vi "Optionen Anzeige zum Speichern_Sicherungskopie.vi"(8 "Optionen":T1 {"SP laden speichern" items=["SP1"=1, "SP2"=2]; "Span Gas Auswahl" items=["1"=1, "2"=2, "3"=3, "4"=4, "5"=5, "6"=6, "7"=7, "8"=8]}, 10 "sichtbar":bool[](array[boolean]), 11 "Optionen (Eingang)":T3) -> (3 "Optionen (Ausgang)":T1 {"SP laden speichern" items=["SP1"=1, "SP2"=2]; "Span Gas Auswahl" items=["1"=1, "2"=2, "3"=3, "4"=4, "5"=5, "6"=6, "7"=7, "8"=8]})   [LabVIEW 2020]
uses:
  System Einstellungen/Optionen.ctl
  Funktionstasten/Spaneingang.ctl
  System Einstellungen/Optionen Eingabe.ctl
  Funktionstasten/Funktionstasten.lvlib
  System Einstellungen/System Einstellungen.lvlib
  System Einstellungen V2.lvlib
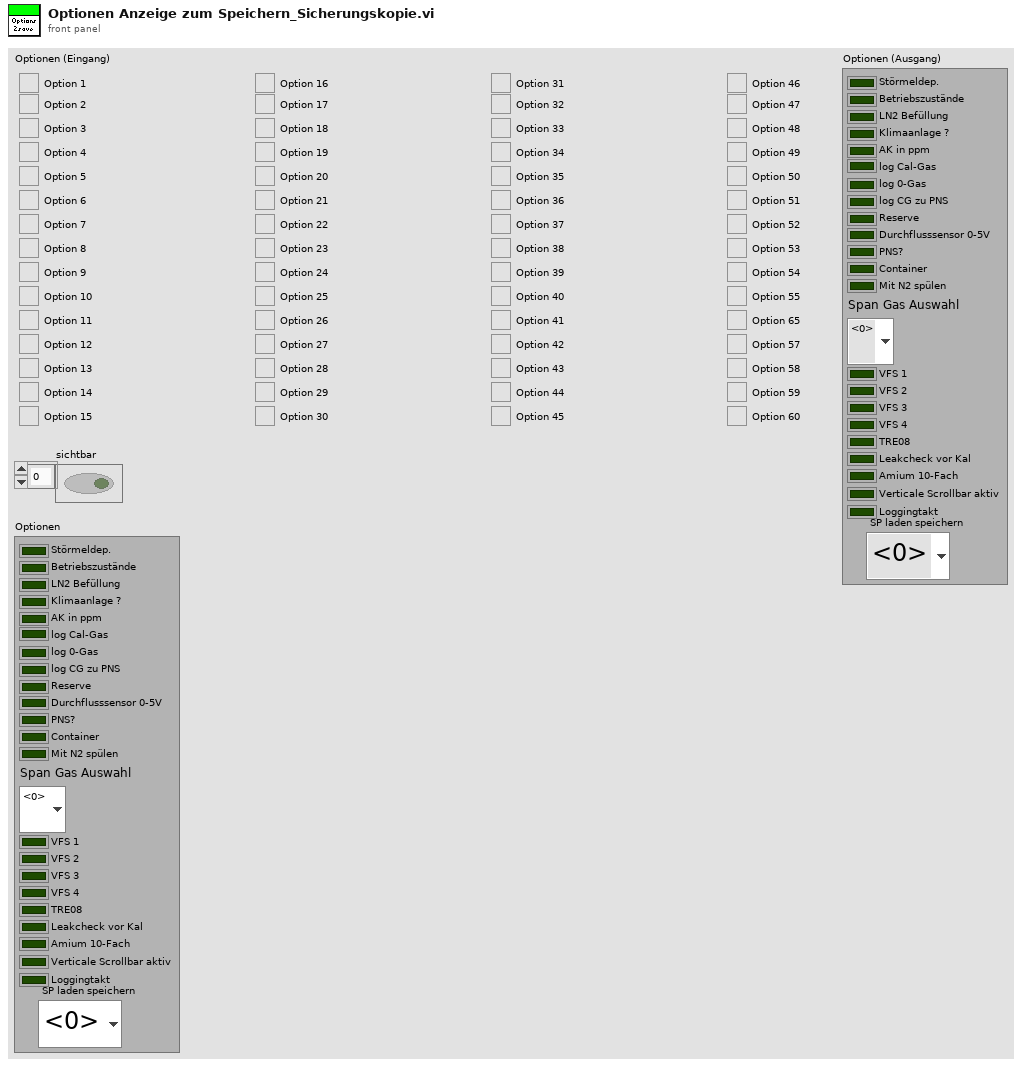
[diagram p1: front panel]
types:
  T1 = typedef "System Einstellungen.lvlib/Optionen.ctl" = cluster{"Störmeldep.":bool, "Betriebszustände":bool, "LN2 Befüllung":bool, "Klimaanlage ?":bool, "AK in ppm":bool, "log Cal-Gas":bool, "log 0-Gas":bool, "log CG zu PNS":bool, "Reserve":bool, "Durchflusssensor 0-5V":bool, "PNS?":bool, "Container":bool, "Mit N2 spülen":bool, "Span Gas Auswahl":T2, "VFS 1":bool, "VFS 2":bool, "VFS 3":bool, "VFS 4":bool, "TRE08":bool, "Leakcheck vor Kal":bool, "Amium 10-Fach":bool, "Verticale Scrollbar aktiv":bool, "Loggingtakt":bool, "SP laden speichern":u16}
  T2 = typedef "Funktionstasten.lvlib/Spaneingang.ctl" = u16
  T3 = typedef "System Einstellungen V2.lvlib/Optionen Eingabe.ctl" = cluster{"Option 1":bool, "Option 2":bool, "Option 3":bool, "Option 4":bool, "Option 5":bool, "Option 6":bool, "Option 7":bool, "Option 8":bool, "Option 9":bool, "Option 10":bool, "Option 11":bool, "Option 12":bool, "Option 13":bool, "Option 14":bool, "Option 15":bool, "Option 16":bool, "Option 17":bool, "Option 18":bool, "Option 19":bool, "Option 20":bool, "Option 21":bool, "Option 22":bool, "Option 23":bool, "Option 24":bool, "Option 25":bool, "Option 26":bool, "Option 27":bool, "Option 28":bool, "Option 29":bool, "Option 30":bool, "Option 31":bool, "Option 32":bool, "Option 33":bool, "Option 34":bool, "Option 35":bool, "Option 36":bool, "Option 37":bool, "Option 38":bool, "Option 39":bool, "Option 40":bool, "Option 41":bool, "Option 42":bool, "Option 43":bool, "Option 44":bool, "Option 45":bool, "Option 46":bool, "Option 47":bool, "Option 48":bool, "Option 49":bool, "Option 50":bool, "Option 51":bool, "Option 52":bool, "Option 53":bool, "Option 54":bool, "Option 55":bool, "Option 56":bool, "Option 57":bool, "Option 58":bool, "Option 59":bool, "Option 60":bool}
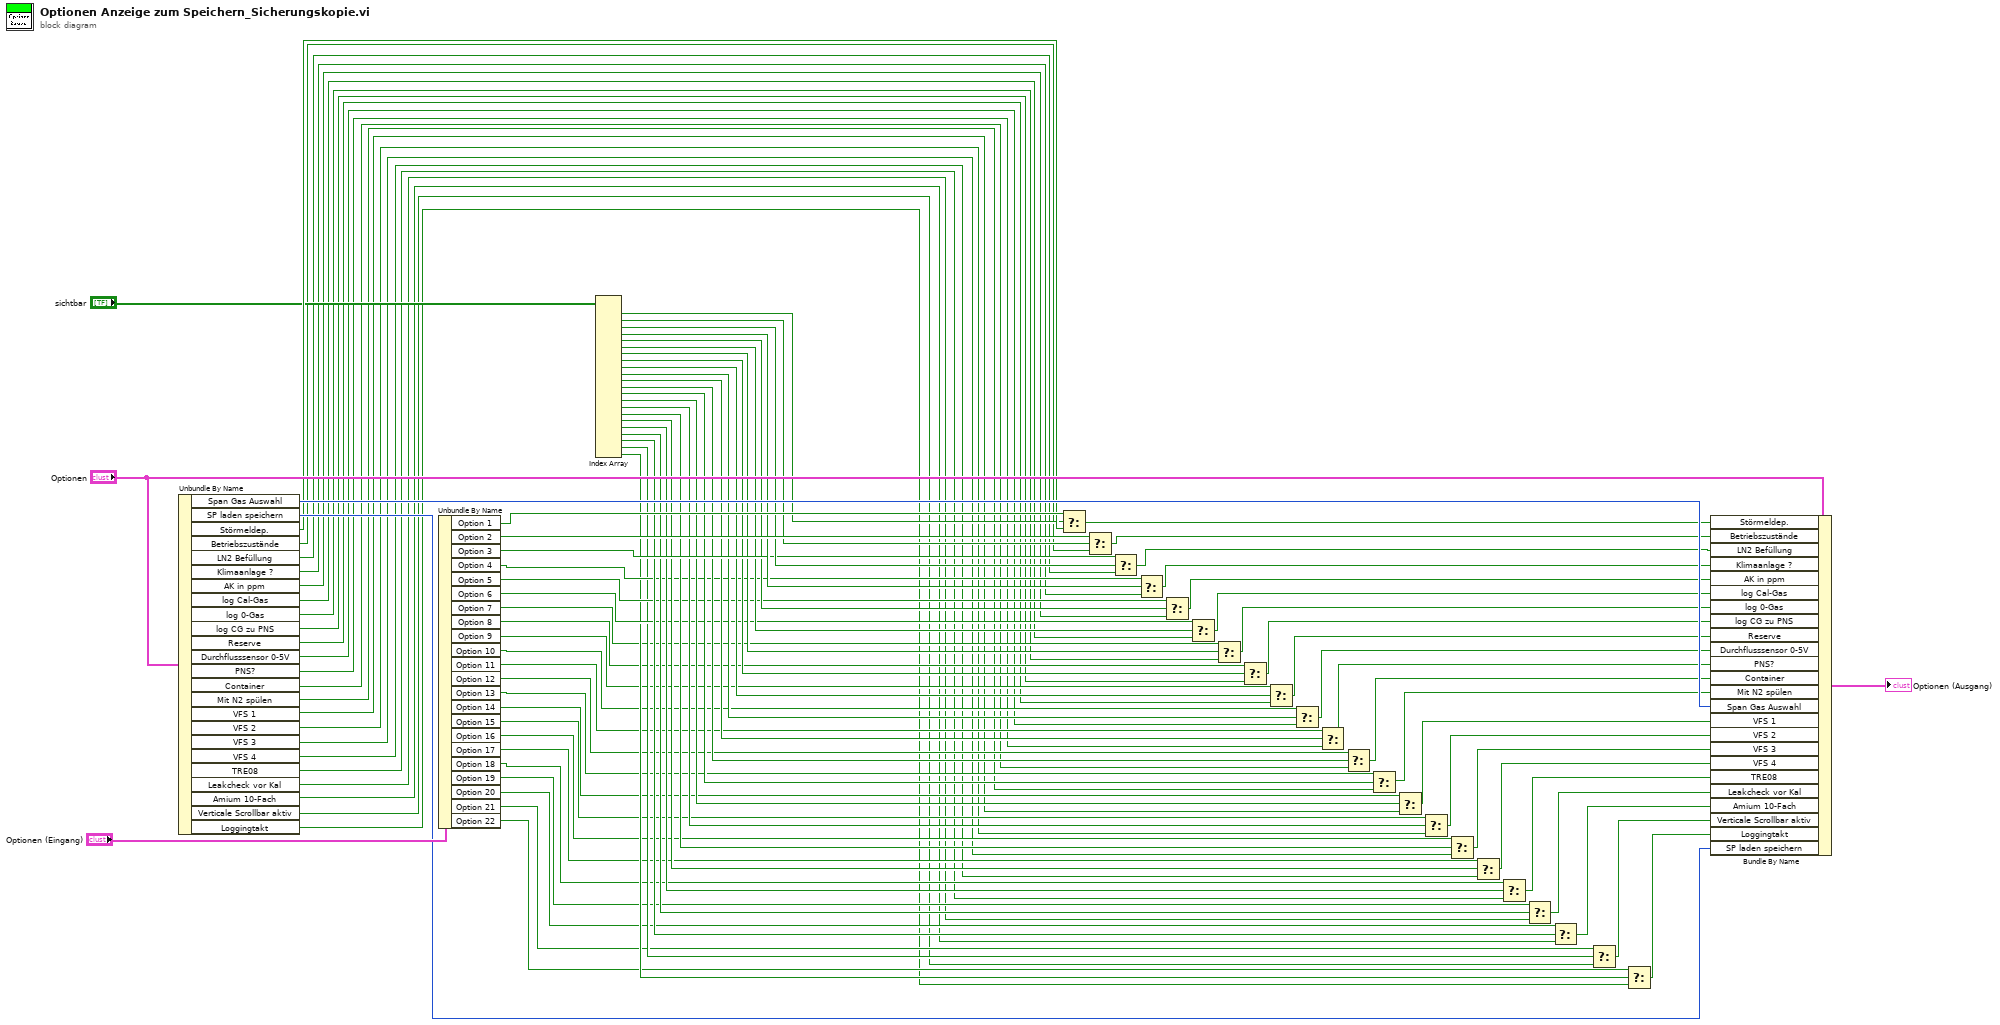
[diagram p0: block diagram]
diagram:
  n1 = Unbundle By Name("Optionen") -> ("Span Gas Auswahl"=w92:T2, "SP laden speichern"=w90:u16, "Störmeldep."=w87:bool, "Betriebszustände"=w11:bool, "LN2 Befüllung"=w78:bool, "Klimaanlage ?"=w58:bool, "AK in ppm"=w57:bool, "log Cal-Gas"=w12:bool, "log 0-Gas"=w33:bool, "log CG zu PNS"=w31:bool, "Reserve"=w29:bool, "Durchflusssensor 0-5V"=w27:bool, "PNS?"=w25:bool, "Container"=w23:bool, "Mit N2 spülen"=w10:bool, "VFS 1"=w9:bool, "VFS 2"=w8:bool, "VFS 3"=w7:bool, "VFS 4"=w6:bool, "TRE08"=w5:bool, "Leakcheck vor Kal"=w4:bool, "Amium 10-Fach"=w3:bool, "Verticale Scrollbar aktiv"=w2:bool, "Loggingtakt"=w1:bool)
  n2 = Unbundle By Name("Optionen (Eingang)") -> ("Option 1"=w88:bool, "Option 2"=w83:bool, "Option 3"=w79:bool, "Option 4"=w61:bool, "Option 5"=w60:bool, "Option 6"=w59:bool, "Option 7"=w34:bool, "Option 8"=w32:bool, "Option 9"=w30:bool, "Option 10"=w28:bool, "Option 11"=w26:bool, "Option 12"=w24:bool, "Option 13"=w22:bool, "Option 14"=w17:bool, "Option 15"=w21:bool, "Option 16"=w20:bool, "Option 17"=w19:bool, "Option 18"=w18:bool, "Option 19"=w16:bool, "Option 20"=w15:bool, "Option 21"=w14:bool, "Option 22"=w13:bool)
  n3 = Index Array(array="sichtbar") -> (element #1=w85:bool, element #2=w82:bool, element #3=w81:bool, element #4=w80:bool, element #5=w77:bool, element #6=w76:bool, element #7=w75:bool, element #8=w74:bool, element #9=w73:bool, element #10=w72:bool, element #11=w71:bool, element #12=w70:bool, element #13=w69:bool, element #14=w68:bool, element #15=w67:bool, element #16=w66:bool, element #17=w65:bool, element #18=w64:bool, element #19=w63:bool, element #20=w62:bool, element #21=w36:bool, element #22=w35:bool)  [unwired: 22 in]
  n4 = Select(t=w88, s=w85, f=w87) -> (s? t:f=w89:bool)
  n5 = Select(t=w83, s=w82, f=w11) -> (s? t:f=w84:bool)
  n6 = Select(t=w79, s=w81, f=w78) -> (s? t:f=w56:bool)
  n7 = Select(t=w61, s=w80, f=w58) -> (s? t:f=w55:bool)
  n8 = Select(t=w60, s=w77, f=w57) -> (s? t:f=w54:bool)
  n9 = Select(t=w59, s=w76, f=w12) -> (s? t:f=w53:bool)
  n10 = Select(t=w34, s=w75, f=w33) -> (s? t:f=w52:bool)
  n11 = Select(t=w32, s=w74, f=w31) -> (s? t:f=w51:bool)
  n12 = Select(t=w30, s=w73, f=w29) -> (s? t:f=w50:bool)
  n13 = Select(t=w28, s=w72, f=w27) -> (s? t:f=w49:bool)
  n14 = Select(t=w26, s=w71, f=w25) -> (s? t:f=w48:bool)
  n15 = Select(t=w24, s=w70, f=w23) -> (s? t:f=w47:bool)
  n16 = Select(t=w22, s=w69, f=w10) -> (s? t:f=w46:bool)
  n17 = Select(t=w17, s=w68, f=w9) -> (s? t:f=w45:bool)
  n18 = Select(t=w21, s=w67, f=w8) -> (s? t:f=w44:bool)
  n19 = Select(t=w20, s=w66, f=w7) -> (s? t:f=w43:bool)
  n20 = Select(t=w19, s=w65, f=w6) -> (s? t:f=w42:bool)
  n21 = Select(t=w18, s=w64, f=w5) -> (s? t:f=w41:bool)
  n22 = Select(t=w16, s=w63, f=w4) -> (s? t:f=w40:bool)
  n23 = Select(t=w15, s=w62, f=w3) -> (s? t:f=w39:bool)
  n24 = Select(t=w14, s=w36, f=w2) -> (s? t:f=w38:bool)
  n25 = Select(t=w13, s=w35, f=w1) -> (s? t:f=w37:bool)
  n26 = Bundle By Name(cluster="Optionen", "Störmeldep."=w89, "Betriebszustände"=w84, "LN2 Befüllung"=w56, "Klimaanlage ?"=w55, "AK in ppm"=w54, "log Cal-Gas"=w53, "log 0-Gas"=w52, "log CG zu PNS"=w51, "Reserve"=w50, "Durchflusssensor 0-5V"=w49, "PNS?"=w48, "Container"=w47, "Mit N2 spülen"=w46, "Span Gas Auswahl"=w92, "VFS 1"=w45, "VFS 2"=w44, "VFS 3"=w43, "VFS 4"=w42, "TRE08"=w41, "Leakcheck vor Kal"=w40, "Amium 10-Fach"=w39, "Verticale Scrollbar aktiv"=w38, "Loggingtakt"=w37, "SP laden speichern"=w90) -> (→"Optionen (Ausgang)":T1)
